vi "UIRefs Full Scale Range.vi"(8 "error in (no error)":errorcluster, 11 "C100L in":refnum<class "C100L.lvclass">) -> (0 "error out":errorcluster, 3 "C100L out":refnum<class "C100L.lvclass">)   [LabVIEW 2021, in "C100L.lvlib" / "C100L.lvclass"]
uses:
  C100L.lvclass
  C100L.lvclass/C100L.ctl
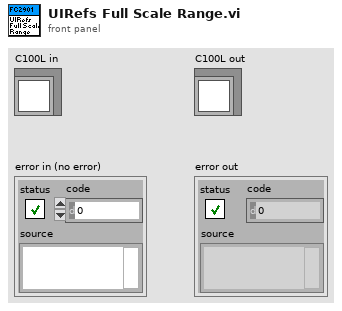
[diagram p1: front panel]
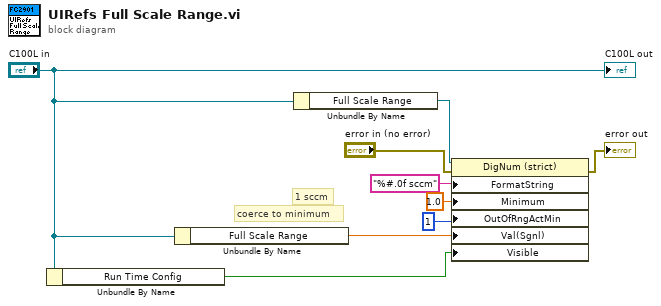
[diagram p0: block diagram]
diagram:
  # "coerce to minimum"
  # "1 sccm"
  n1 = Unbundle By Name("C100L in") -> ("Run Time Config"=w3:bool)
  n2 = Unbundle By Name("C100L in") -> ("Full Scale Range"=w5:dbl)
  n3 = Unbundle By Name("C100L in") -> ("Full Scale Range"=w9:refnum<vi>)
  n4 = property class="DigNum (strict)"(reference=w9, error in="error in (no error)", "FormatString"="%#.0f sccm" ("Format String"), "Minimum"=1.0 ("Data Entry Limits:Minimum"), "OutOfRngActMin"=u8 1 ("Response to Value Outside Limits:Minimum"), "Val(Sgnl)"=w5, "Visible"=w3) -> (error out=→"error out":errorcluster)  [unwired: 1 out]
  "C100L out" <- "C100L in"
